vi "Data logger Scalar Enqueue Function.vi"(0 "QRef in":refnum<queue>, 5 "Q1 Message":T1={"state"=enum."Idle", "data"=variant}, 11 "Error in":errorcluster, 13 "Mode":enum16{"Back", "Front", "Replace"}(ring)) -> (4 "QRef out":refnum<queue>, 15 "Error out":errorcluster)   [LabVIEW 2014]
uses:
  TypeDef/Q1 Message.ctl
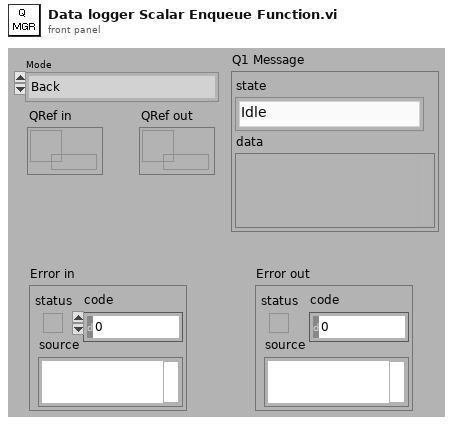
[diagram p1: front panel]
types:
  T1 = typedef "Q1 Message.ctl" = cluster{"state":enum16{"initialize 1", "initialize 2", "initialize 3", "initialize 4", "initialize 5", "initialize 6", "initialize 7", "initialize 8", "initialize 9", "Idle", "Preparation 1", "Preparation 2", "Preparation 3", "Preparation 4", "Record", "Stop recording", "Exit", "Defrag", "View", "Create Database", "Update folder setting", "Update Preference", "Update TDMS properties", "CSV Delimiter", "DB Type", "Hidden Processes", "Replace Database", "Logged File Viewer", "Defrag Prompt File", "View Prompt File", "Save to config file", "Open from config file"}, "data":variant}
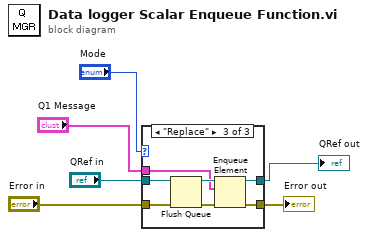
[diagram p0: block diagram]
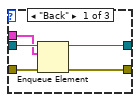
[diagram p2: hidden frame]
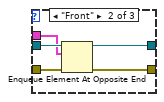
[diagram p3: hidden frame]
diagram:
  n1 = case shown="\"Replace\"" "Mode" {
    tunnel: "Q1 Message" -> [w9 w12 w21]
    tunnel: "QRef in" -> [w11 w16 w23]
    tunnel: [w10 w15 w20] -> w2
    tunnel: "Error in" -> [w8 w14 w18]
    tunnel: [w7 w13 w17] -> w6
    frame "Back" {
      n2 = Enqueue Element(queue=w11, element=w9, error in (no error)=w8) -> (queue out=w10:refnum<queue>, error out=w7:errorcluster)  [unwired: 1 in, 1 out]
    }
    frame "Front" {
      n3 = Enqueue Element At Opposite End(queue=w16, element=w12, error in (no error)=w14) -> (queue out=w15:refnum<queue>, error out=w13:errorcluster)  [unwired: 1 in, 1 out]
    }
    frame "Replace" {
      n4 = Flush Queue(queue=w23, error in (no error)=w18) -> (queue out=w22:refnum<queue>, error out=w19:errorcluster)  [unwired: 1 out]
      n5 = Enqueue Element(queue=w22, element=w21, error in (no error)=w19) -> (queue out=w20:refnum<queue>, error out=w17:errorcluster)  [unwired: 1 in, 1 out]
    }
  }
  "Error out" <- w6
  "QRef out" <- w2
